vi "ReadGyro.vi"   [LabVIEW 2016, in "Moving Motor.lvrbt"]
uses:
  Moving Motor.lvrbt
  <vilib>/NXT/HiTechnic/HiTechnic Controls/HiTechnic Port.ctl
  <vilib>/NXT/Block Support/NXT_InputPort.ctl
  <vilib>/NXT/Hardware/Plugins/Tetrix DC Motor/TetrixDCMotorAddress.ctl
  <vilib>/NXT/Dual Mode Library/Waits/Wait_Num.vi
  <vilib>/NXT/Dual Mode Library/Waits/Wait_Num(msec).vi
  <vilib>/NXT/Dual Mode Library/Sensors/Read_Timer.vi
  <vilib>/NXT/Dual Mode Library/prims/sign/sign_int.vi
  <vilib>/NXT/NXTIO Xnodes/NXTIONodeSubVIs/TETRIX IO Move DC Motors.vi
  <vilib>/NXT/NXTIO Xnodes/NXTIONodeSubVIs/LEGOStopAllMotors.vi
  <vilib>/NXT/NXTIO Xnodes/AddressXNode/NXTIOAddress.xnode
  <vilib>/NXT/NXTIO Xnodes/NXTIOXNode/NXTIO.xnode
  <vilib>/NXT/Subs/LVHSConnector.ctl
  <vilib>/NXT/LegoClasses/BrickReference/BrickReference.lvclass
types:
  T1 = typedef "HiTechnic Port.ctl" = cluster{"Port":T2, "MUX Port":u8}
  T2 = typedef "NXT_InputPort.ctl" = u32
  T3 = typedef "LVHSConnector.ctl" = refnum<class "BrickReference.lvclass">
  T4 = typedef "TetrixDCMotorAddress.ctl" = i32
  T5 = cluster{"TetrixDCMotor":T4, "TetrixDCMotor 2":T4}
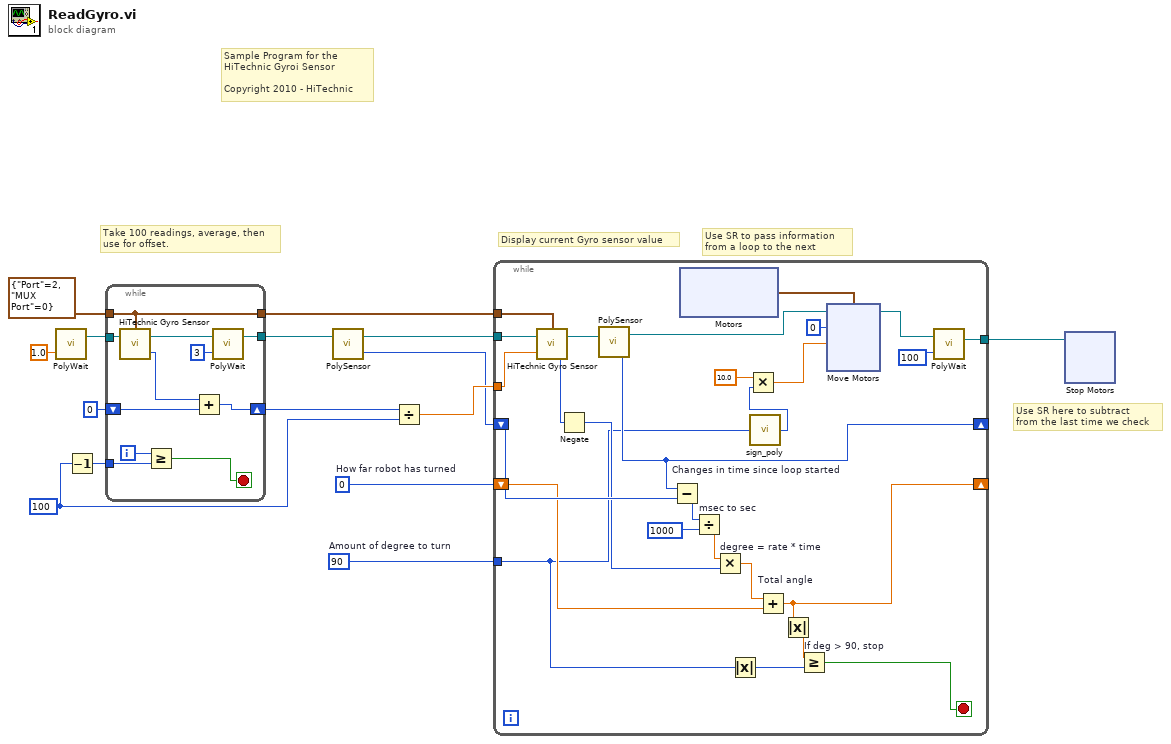
[diagram p0: block diagram]
diagram:
  w5 = 0  # How far robot has turned
  w6 = 90  # Amount of degree to turn
  w12 = i16 100
  # "Use SR here to subtract\nfrom the last time we check"
  # "Use SR to pass information \nfrom a loop to the next"
  # "Display current Gyro sensor value"
  # "Take 100 readings, average, then\nuse for offset."
  # "Sample Program for the\nHiTechnic Gyroi Sensor\n\nCopyright 2010 - HiTechnic"
  n1 = call-poly <vilib>:"PolyWait.vi"("Time (1 sec)"=sgl 1.0 ("Time (sec)")) -> ("NXT/EV3"=w8:T3)  [unwired: 3 in]
  n2 = Decrement(x=w12) -> (x-1=w14:i16)
  n3 = while {
    shift-right: [w24] -> w13
    shift-left: 0 -> [w25]
    tunnel: w14 -> [w22]
    tunnel: [w20] -> w4
    tunnel: T1 {"Port"=2, "MUX Port"=0} ("Port/MUX") -> [w17]
    tunnel: [w17] -> w9
    tunnel: w8 -> [w16]
    i -> [w23]
    stop <- w21 stop-if-true
    n4 = call <vilib>:"HiTechnic Gyro Sensor.vi"("NXT/EV3"=w16, "Port/MUX"=w17) -> ("Gyro Value"=w26:i16, "NXT/EV3"=w18:T3)  [unwired: 1 in]
    n5 = Greater Or Equal?(x=w23, y=w22) -> (x >= y?=w21:bool)
    n6 = Add(x=w26, y=w25) -> (x+y=w24:i32)
    n7 = call-poly <vilib>:"PolyWait.vi"("Time (100 msec)"=u32 3 ("Time (sec)"), "NXT/EV3"=w18) -> ("NXT/EV3"=w20:T3)  [unwired: 2 in]
  }
  n8 = call-poly <vilib>:"PolySensor.vi"("NXT/EV3"=w4) -> ("Value (msec)"=w2:u32, "NXT/EV3"=w3:T3)  [unwired: 2 in]
  n9 = Divide(x=w13, y=w12) -> (x/y=w11:dbl)
  n10 = while {
    tunnel: w11 -> [w53]
    tunnel: w9 -> [w52]
    tunnel: w6 -> [w33]
    shift-right: [w41] -> _
    shift-left: w5 -> [w42]
    tunnel: w3 -> [w50]
    shift-right: [w45] -> _
    shift-left: w2 -> [w48]
    tunnel: [w27] -> w1
    stop <- w40 stop-if-true
    n11 = call <vilib>:"HiTechnic Gyro Sensor.vi"("Offset"=w53, "NXT/EV3"=w50, "Port/MUX"=w52) -> ("Gyro Value"=w39:i16, "NXT/EV3"=w49:T3)
    n12 = Negate(x=w39) -> (-x=w38:i16)
    n13 = call-poly <vilib>:"PolySensor.vi"("NXT/EV3"=w49) -> ("Value (msec)"=w45:u32, "NXT/EV3"=w31:T3)  [unwired: 2 in]
    n14 = Subtract "Changes in time since loop started"(x=w45, y=w48) -> (x-y=w47:u32)
    n15 = xnode "Motors"() -> ("Motor"=w32:cluster{"TetrixDCMotor":T4, "TetrixDCMotor":T4})
    n16 = Divide "msec to sec"(x=w47, y=1000) -> (x/y=w44:dbl)
    n17 = Multiply "degree = rate * time"(x=w44, y=w38) -> (x*y=w43:dbl)
    n18 = Absolute Value(x=w33) -> (abs(x)=w36:i32)
    n19 = call-poly <vilib>:"sign_poly.vi"("number"=w33) -> ("-1, 0, 1"=w34:i32)  [unwired: 4 in]
    n20 = Multiply(x=10.0, y=w34) -> (x*y=w29:dbl)
    n21 = Add "Total angle"(x=w43, y=w42) -> (x+y=w41:dbl)
    n22 = Absolute Value(x=w41) -> (abs(x)=w37:dbl)
    n23 = Greater Or Equal? "If deg > 90, stop"(x=w37, y=w36) -> (x >= y?=w40:bool)
    n24 = xnode "Move Motors"("Power/Speed 2"=w29, "Power/Speed 1"=i8 0, "Motors"=w32, "NXT/EV3"=w31) -> ("NXT/EV3"=w30:T3)
    n25 = call-poly <vilib>:"PolyWait.vi"("Time (100 msec)"=u32 100 ("Time (sec)"), "NXT/EV3"=w30) -> ("NXT/EV3"=w27:T3)  [unwired: 2 in]
  }
  n26 = xnode "Stop Motors"("NXT/EV3"=w1) -> ()  [unwired: 1 in, 1 out]
